vi "Laser-Unit-Converter.vi"() -> ()   [LabVIEW 2018]
panel:
  out "nm":dbl
  in  "Input Units?":bool
  out "cm-1":dbl
  in  "Input":dbl=220.1
  # "cm-1"
  # "nm"
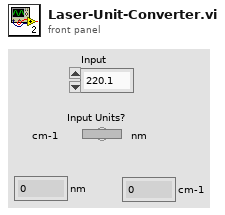
[diagram p1: front panel]
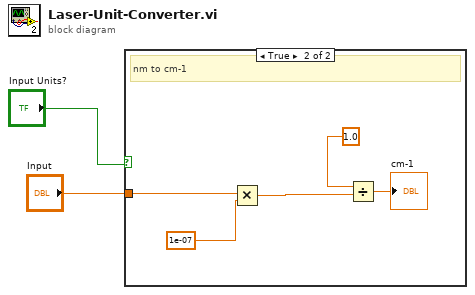
[diagram p0: block diagram]
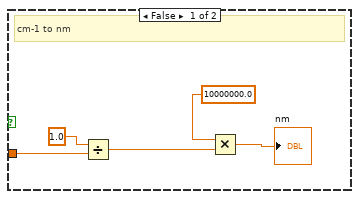
[diagram p2: hidden frame]
diagram:
  n1 = case shown="True" "Input Units?" {
    tunnel: "Input" -> [w7 w11]
    frame False {
      # "cm-1 to nm"
      n2 = Divide(x=1.0, y=w7) -> (x/y=w5:dbl)
      n3 = Multiply(x=10000000.0, y=w5) -> (x*y=→"nm":dbl)
    }
    frame True {
      # "nm to cm-1"
      n4 = Multiply(x=w11, y=1e-07) -> (x*y=w10:dbl)
      n5 = Divide(x=1.0, y=w10) -> (x/y=→"cm-1":dbl)
    }
  }
